vi "N Channel 1 Sample - Manual Timestamp.vi"() -> ()   [LabVIEW 2026]
uses:
  <userlib>/Synnax/synnax_lib.lvlibp/typedefs/connection_config.ctl
  <userlib>/Synnax/synnax_lib.lvlibp/classes/Client/Private/synnax channel retrieve keys Array.vi
  <userlib>/Synnax/synnax_lib.lvlibp/classes/Writer/Private/synnax writer open Array.vi
  <userlib>/Synnax/synnax_lib.lvlibp/classes/Writer/Private/Writes/I32/Write NCh 1Samp (I32).vi
  <userlib>/Synnax/synnax_lib.lvlibp/classes/Client/Synnax Client.lvclass
  <userlib>/Synnax/synnax_lib.lvlibp/classes/Synnax Writer.lvclass
  <userlib>/Synnax/synnax_lib.lvlibp
panel:
  out "error out":errorcluster
  in  "Channels":string[](array[numeric])=["my_i32_idx", "my_i32_ch1", "my_i32_ch2", "my_i32_ch3", "my_i32_ch4"]
  in  "Stop":bool
  in  "Connection Config":T1={"host"="localhost", "port"=9090, "username"="synnax", "password"="seldon"}
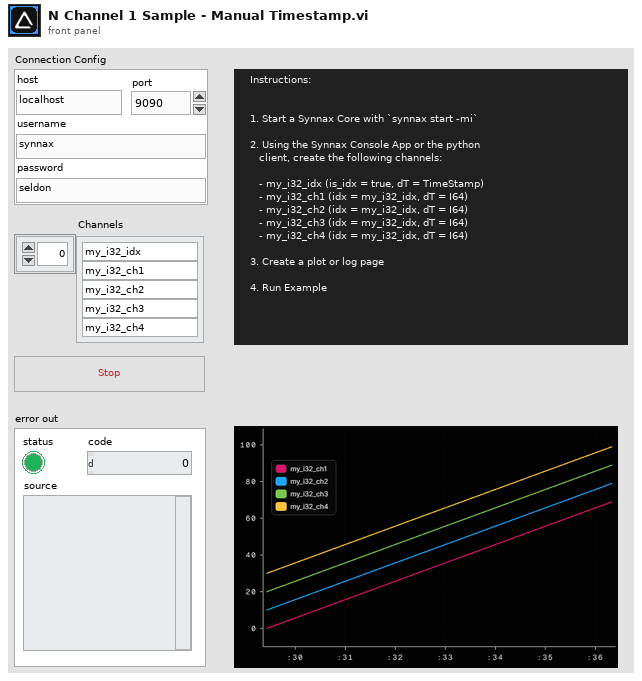
[diagram p1: front panel]
types:
  T1 = typedef "synnax_lib.lvlibp/connection_config.ctl" = cluster{"host":string, "port":u16, "username":string, "password":string}
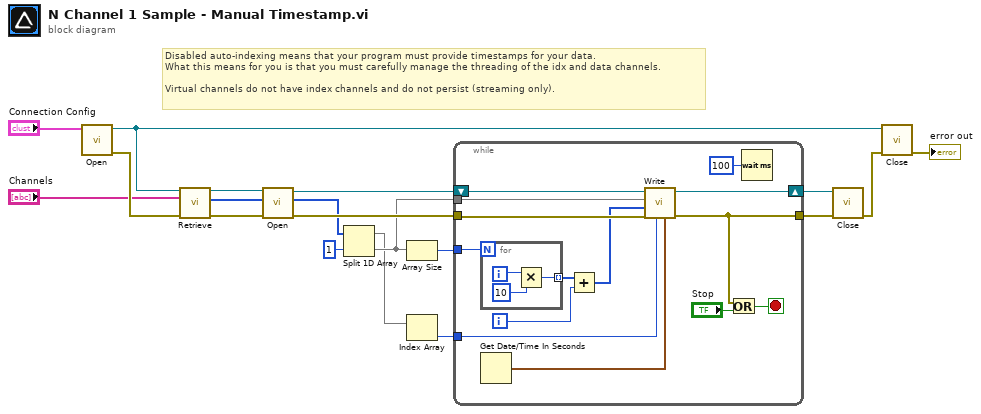
[diagram p0: block diagram]
diagram:
  # "Disabled auto-indexing means that your program must provide timestamps for your data.\nWhat this means for you is that you must carefully manage the threading of the idx and data channels.\n\nVirtual channels do not have index channels and do not persist (streaming only)."
  n1 = call <userlib>:"Open.vi"("Connection Config"="Connection Config") -> ("error out"=w14:errorcluster, "Synnax Client out"=w16:refnum<class "Synnax Client.lvclass">)  [unwired: 9 in]
  n2 = call-poly <userlib>:"Retrieve.vi"("Synnax Client in"=w16, "channel names"="Channels", "error in"=w14) -> ("Synnax Client out"=w10:refnum<class "Synnax Client.lvclass">, "channel keys"=w9:u32[], "error out"=w18:errorcluster)  [unwired: 8 in, 2 out]
  n3 = call-poly <userlib>:"Open.vi"("error in"=w18, "channels in"=w9, "Synnax Client in"=w10) -> ("error out"=w11:errorcluster, "channels out"=w7:u32[], "writer out"=w13:refnum<class "Synnax Writer.lvclass">)  [unwired: 6 in]
  n4 = Split 1D Array(array=w7, index=1) -> (first subarray=w3:u32[], second subarray=w5:u32[])
  n5 = Array Size(array=w5) -> (size(s)=w4:i32)
  n6 = Index Array(array=w3) -> (element=w2:u32)  [unwired: 1 in]
  n7 = while {
    shift-right: [w32] -> w12
    shift-left: w13 -> [w33]
    tunnel: w11 -> [w31]
    tunnel: [w20] -> w19
    tunnel: w5 -> [w27]
    tunnel: w4 -> [w26]
    tunnel: w2 -> [w23]
    i -> [w24]
    stop <- w21 stop-if-true
    n8 = for {
      N: w26 -> [_]
      tunnel: [w35] -> w29 mode=indexing
      i -> [w36]
      n9 = Multiply(x=w36, y=10) -> (x*y=w35:i32)
    }
    n10 = Get Date/Time In Seconds() -> (seconds since 1Jan1904=w22:timestamp)
    n11 = Add(x=w29, y=w24) -> (x+y=w25:i32[])
    n12 = call-poly <userlib>:"Write.vi"("timestamp"=w22, "index_channel"=w23, "error in"=w31, "data"=w25, "channels"=w27, "Writer"=w33) -> ("error out"=w20:errorcluster, "Writer Out"=w32:refnum<class "Synnax Writer.lvclass">)  [unwired: 4 in]
    n13 = Or(x=w20, y="Stop") -> (x .or. y?=w21:bool)
    n14 = Wait (ms)(milliseconds to wait=u32 100) -> ()  [unwired: 1 out]
  }
  n15 = call <userlib>:"Close.vi"("error in"=w19, "writer"=w12) -> ("error out"=w15:errorcluster)  [unwired: 9 in]
  n16 = call <userlib>:"Close.vi"("error in"=w15, "Synnax Client in"=w16) -> ("error out"=→"error out":errorcluster)  [unwired: 9 in]
